vi "ChirpOOP_V1.vi"() -> ()   [LabVIEW 2014, in "ChirpEIS.lvclass"]
uses:
  ChirpEIS.lvclass
  States.ctl
  ChirpEIS.lvclass/ChirpEIS.ctl
panel:
  out "Chirp Control.sampling Info":cluster{"Fs":dbl, "#s":dbl}
  out "Experiment Variables.Duration":dbl
  out "Experiment Variables.StartFreq":dbl
  out "error out":errorcluster
  in  "Chirp control":T1={"R external(Ohm)"=96.0, "Chirp Start(Hz)"=0.1, "Chirp Ends(Hz)"=10.0, "Vmin"=0.0, "VInc"=0.2, "Vmax"=0.8, "Chirp T(s)"=0.8}
  out "data 2":dynamicdata(graph) caption="data"
  in  "stop":bool
  out "State":T2=enum."IncreaseVoltage"
  out "DC bias":dbl
  in  "Path":path=path "C:/Users/YuanYuan/Desktop/Labview Data/Chirp2"
  in  "Setup":string="TOKIN1"
  in  "ChirpEIS.lvclass":refnum<class "ChirpEIS.lvclass">
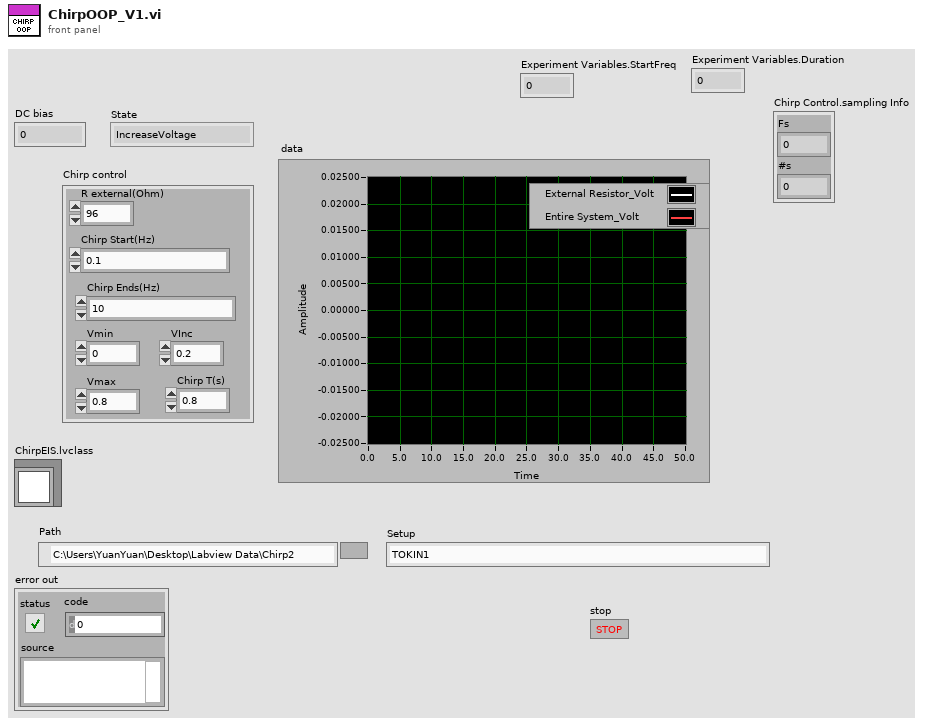
[diagram p1: front panel]
types:
  T1 = cluster{"R external(Ohm)":dbl, "Chirp Start(Hz)":dbl, "Chirp Ends(Hz)":dbl, "Vmin":dbl, "VInc":dbl, "Vmax":dbl, "Chirp T(s)":dbl}
  T2 = typedef "States.ctl" = enum16{"AddDuration", "AddFreq", "CreateNewFile", "Wait", "IncreaseVoltage", "DFT", "ChirpMeasurement", "Initialize", "Ternimate"}
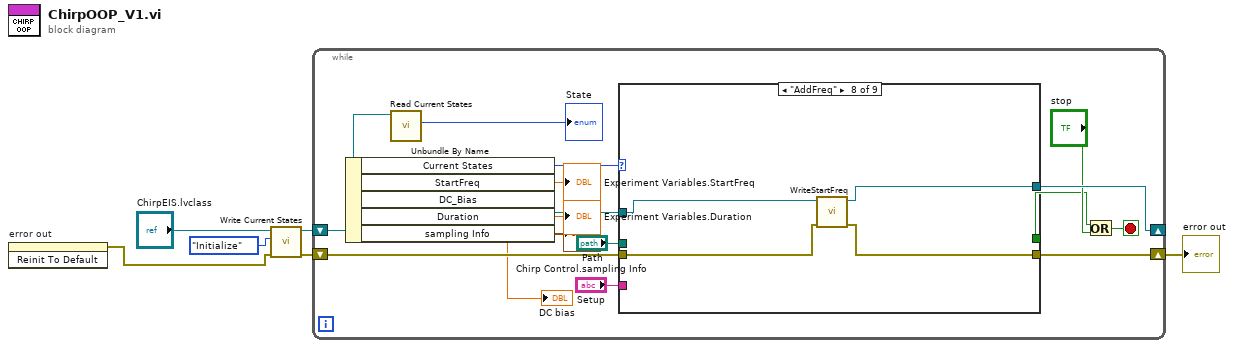
[diagram p0: block diagram]
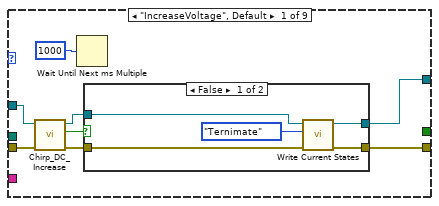
[diagram p2: hidden frame]
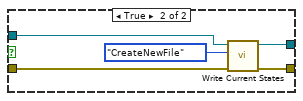
[diagram p3: hidden frame]
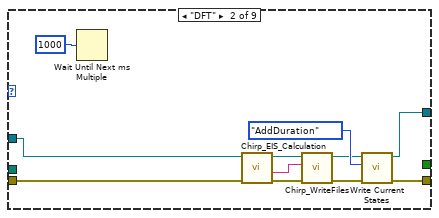
[diagram p4: hidden frame]
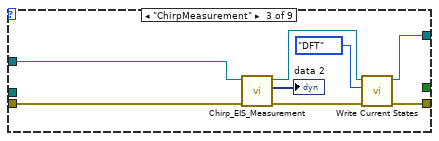
[diagram p5: hidden frame]
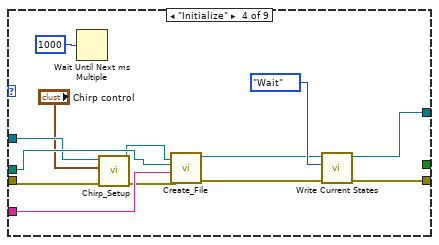
[diagram p6: hidden frame]
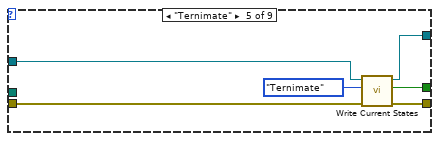
[diagram p7: hidden frame]
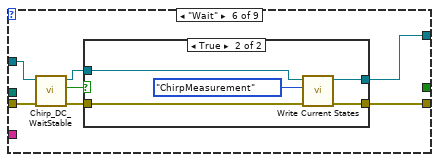
[diagram p8: hidden frame]
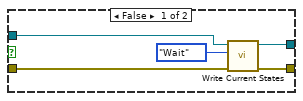
[diagram p9: hidden frame]
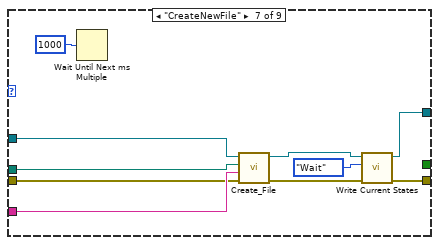
[diagram p10: hidden frame]
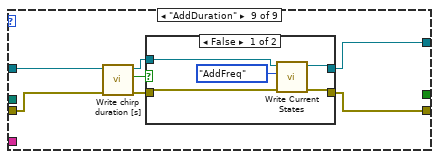
[diagram p11: hidden frame]
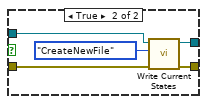
[diagram p12: hidden frame]
diagram:
  n1 = invoke on="error out" class="Clust (strict)" method="Reinit To Default"() -> (error out=w1:errorcluster)  [unwired: 3 in, 2 out]
  n2 = call-dynamic "Write Current States.vi"("error in (no error)"=w1, "Enum"=States."Initialize", "ChirpEIS in"="ChirpEIS.lvclass") -> ("error out"=w3:errorcluster, "ChirpEIS out"=w5:refnum<class "ChirpEIS.lvclass">)  [unwired: 6 in, 1 out]
  n3 = while {
    shift-right: [w19] -> _
    shift-left: w5 -> [w17]
    shift-right: [w18] -> w2
    shift-left: w3 -> [w20]
    stop <- w13 stop-if-true
    n4 = Unbundle By Name(w17) -> ("Current States"=w21:T2, "StartFreq"=→"Experiment Variables.StartFreq":dbl, "DC_Bias"=→"DC bias":dbl, "Duration"=→"Experiment Variables.Duration":dbl, "sampling Info"=→"Chirp Control.sampling Info":cluster{"Fs":dbl, "#s":dbl})
    n5 = call-dynamic "Read Current States.vi"("ChirpEIS in"=w17) -> ("Enum"=→"State":T2)  [unwired: 8 in, 2 out]
    n6 = case shown="\"AddFreq\"" w21 {
      tunnel: w17 -> [w26 w47 w51 w65 w77 w81 w102 w108 w115]
      tunnel: w20 -> [w23 w46 w55 w64 w76 w80 w101 w107 w114]
      tunnel: [w29 w49 w57 w70 w75 w84 w100 w106 w110] -> w19
      tunnel: [w28 w48 w56 w69 w74 w83 w99 w105 w109] -> w18
      tunnel: [_ _ _ _ w72 _ _ _ _] -> w14
      tunnel: "Path" -> [_ _ _ w68 _ _ w104 _ _]
      tunnel: "Setup" -> [_ _ _ w67 _ _ w103 _ _]
      frame "IncreaseVoltage", Default {
        n7 = call-dynamic "Chirp_DC_Increase.vi"("error in (no error)"=w23, "ChirpEIS in"=w26) -> ("error out"=w24:errorcluster, "Less than Max DC"=w27:bool, "ChirpEIS out"=w25:refnum<class "ChirpEIS.lvclass">)  [unwired: 7 in]
        n8 = Wait Until Next ms Multiple(millisecond multiple=u32 1000) -> ()  [unwired: 1 out]
        n9 = case shown="False" w27 {
          tunnel: w25 -> [w31 w39]
          tunnel: w24 -> [w30 w38]
          tunnel: [w33 w37] -> w29
          tunnel: [w32 w36] -> w28
          frame False {
            n10 = call-dynamic "Write Current States.vi"("error in (no error)"=w30, "Enum"=States."Ternimate", "ChirpEIS in"=w31) -> ("error out"=w32:errorcluster, "ChirpEIS out"=w33:refnum<class "ChirpEIS.lvclass">)  [unwired: 6 in, 1 out]
          }
          frame True {
            n11 = call-dynamic "Write Current States.vi"("error in (no error)"=w38, "Enum"=States."CreateNewFile", "ChirpEIS in"=w39) -> ("error out"=w36:errorcluster, "ChirpEIS out"=w37:refnum<class "ChirpEIS.lvclass">)  [unwired: 6 in, 1 out]
          }
        }
      }
      frame "DFT" {
        n12 = Wait Until Next ms Multiple(millisecond multiple=u32 1000) -> ()  [unwired: 1 out]
        n13 = call-dynamic "Chirp_EIS_Calculation.vi"("error in (no error)"=w46, "ChirpEIS in"=w47) -> ("error out"=w43:errorcluster, "EIS Results"=w45:string, "ChirpEIS out"=w44:refnum<class "ChirpEIS.lvclass">)  [unwired: 6 in, 1 out]
        n14 = call-dynamic "Chirp_WriteFiles.vi"("error in (no error)"=w43, "Data"=w45, "ChirpEIS in"=w44) -> ("error out"=w41:errorcluster, "ChirpEIS out"=w42:refnum<class "ChirpEIS.lvclass">)  [unwired: 7 in]
        n15 = call-dynamic "Write Current States.vi"("error in (no error)"=w41, "Enum"=States."AddDuration", "ChirpEIS in"=w42) -> ("error out"=w48:errorcluster, "ChirpEIS out"=w49:refnum<class "ChirpEIS.lvclass">)  [unwired: 6 in, 1 out]
      }
      frame "ChirpMeasurement" {
        n16 = call-dynamic "Chirp_EIS_Measurement.vi"("error in (no error)"=w55, "ChirpEIS in"=w51) -> ("error out"=w53:errorcluster, "data"=→"data 2":dynamicdata, "ChirpEIS out"=w54:refnum<class "ChirpEIS.lvclass">)  [unwired: 5 in, 2 out]
        n17 = call-dynamic "Write Current States.vi"("error in (no error)"=w53, "Enum"=States."DFT", "ChirpEIS in"=w54) -> ("error out"=w56:errorcluster, "ChirpEIS out"=w57:refnum<class "ChirpEIS.lvclass">)  [unwired: 6 in, 1 out]
      }
      frame "Initialize" {
        n18 = Wait Until Next ms Multiple(millisecond multiple=u32 1000) -> ()  [unwired: 1 out]
        n19 = call "Chirp_Setup.vi"("error in (no error)"=w64, "Chirp control"="Chirp control", "ChirpEIS in"=w65) -> ("error out"=w62:errorcluster, "ChirpEIS out"=w63:refnum<class "ChirpEIS.lvclass">)  [unwired: 7 in]
        n20 = call "Create_File.vi"("error in (no error)"=w62, "Setup"=w67, "Path"=w68, "ChirpEIS in"=w63) -> ("error out"=w59:errorcluster, "ChirpEIS out"=w60:refnum<class "ChirpEIS.lvclass">)  [unwired: 6 in]
        n21 = call-dynamic "Write Current States.vi"("error in (no error)"=w59, "Enum"=States."Wait", "ChirpEIS in"=w60) -> ("error out"=w69:errorcluster, "ChirpEIS out"=w70:refnum<class "ChirpEIS.lvclass">)  [unwired: 6 in, 1 out]
      }
      frame "Ternimate" {
        n22 = call-dynamic "Write Current States.vi"("error in (no error)"=w76, "Enum"=States."Ternimate", "ChirpEIS in"=w77) -> ("error out"=w74:errorcluster, "Boolean"=w72:bool, "ChirpEIS out"=w75:refnum<class "ChirpEIS.lvclass">)  [unwired: 6 in]
      }
      frame "Wait" {
        n23 = call-dynamic "Chirp_DC_WaitStable.vi"("error in (no error)"=w80, "ChirpEIS in"=w81) -> ("error out"=w78:errorcluster, "logical AND"=w82:bool, "ChirpEIS out"=w79:refnum<class "ChirpEIS.lvclass">)  [unwired: 6 in, 1 out]
        n24 = case shown="True" w82 {
          tunnel: w79 -> [w86 w94]
          tunnel: w78 -> [w85 w93]
          tunnel: [w88 w92] -> w84
          tunnel: [w87 w91] -> w83
          frame False {
            n25 = call-dynamic "Write Current States.vi"("error in (no error)"=w85, "Enum"=States."Wait", "ChirpEIS in"=w86) -> ("error out"=w87:errorcluster, "ChirpEIS out"=w88:refnum<class "ChirpEIS.lvclass">)  [unwired: 6 in, 1 out]
          }
          frame True {
            n26 = call-dynamic "Write Current States.vi"("error in (no error)"=w93, "Enum"=States."ChirpMeasurement", "ChirpEIS in"=w94) -> ("error out"=w91:errorcluster, "ChirpEIS out"=w92:refnum<class "ChirpEIS.lvclass">)  [unwired: 6 in, 1 out]
          }
        }
      }
      frame "CreateNewFile" {
        n27 = Wait Until Next ms Multiple(millisecond multiple=u32 1000) -> ()  [unwired: 1 out]
        n28 = call "Create_File.vi"("error in (no error)"=w101, "Setup"=w103, "Path"=w104, "ChirpEIS in"=w102) -> ("error out"=w97:errorcluster, "ChirpEIS out"=w98:refnum<class "ChirpEIS.lvclass">)  [unwired: 6 in]
        n29 = call-dynamic "Write Current States.vi"("error in (no error)"=w97, "Enum"=States."Wait", "ChirpEIS in"=w98) -> ("error out"=w99:errorcluster, "ChirpEIS out"=w100:refnum<class "ChirpEIS.lvclass">)  [unwired: 6 in, 1 out]
      }
      frame "AddFreq" {
        n30 = call-dynamic "WriteStartFreq.vi"("error in (no error)"=w107, "ChirpEIS in"=w108) -> ("error out"=w105:errorcluster, "ChirpEIS out"=w106:refnum<class "ChirpEIS.lvclass">)  [unwired: 8 in]
      }
      frame "AddDuration" {
        n31 = call-dynamic "Write chirp duration [s].vi"("error in (no error)"=w114, "ChirpEIS in"=w115) -> ("error out"=w112:errorcluster, "Less than Max"=w111:bool, "ChirpEIS out"=w113:refnum<class "ChirpEIS.lvclass">)  [unwired: 7 in]
        n32 = case shown="False" w111 {
          tunnel: w113 -> [w118 w125]
          tunnel: w112 -> [w117 w124]
          tunnel: [w120 w123] -> w110
          tunnel: [w119 w122] -> w109
          frame False {
            n33 = call-dynamic "Write Current States.vi"("error in (no error)"=w117, "Enum"=States."AddFreq", "ChirpEIS in"=w118) -> ("error out"=w119:errorcluster, "ChirpEIS out"=w120:refnum<class "ChirpEIS.lvclass">)  [unwired: 6 in, 1 out]
          }
          frame True {
            n34 = call-dynamic "Write Current States.vi"("error in (no error)"=w124, "Enum"=States."CreateNewFile", "ChirpEIS in"=w125) -> ("error out"=w122:errorcluster, "ChirpEIS out"=w123:refnum<class "ChirpEIS.lvclass">)  [unwired: 6 in, 1 out]
          }
        }
      }
    }
    n35 = Or(x=w14, y="stop") -> (x .or. y?=w13:bool)
  }
  "error out" <- w2
